vi "mxwScript_API_SetVal_Blob.vi"(7 "itemSelectType":T1, 8 "error in (no error)":errorcluster, 9 "blob":variant, 10 "label":string, 11 "index":i32) -> (0 "error out":errorcluster, 3 "parameter":T2)   [LabVIEW 2017]
uses:
  codeGenAPISupport.llb/cgAPI_mxwScript_Parameter.ctl
  codeGenAPISupport.llb/cgAPI_mxwScript_SetParm_ItemSelectType.ctl
  codeGenAPISupport.llb/cgAPI_mxwScript_SetParm_BlobN.ctl
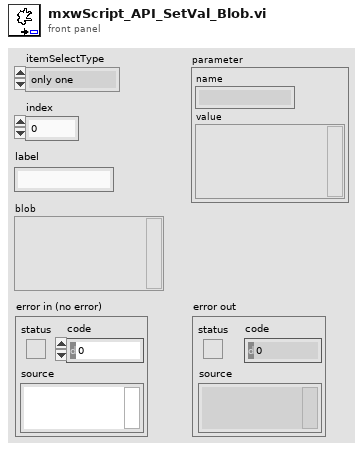
[diagram p1: front panel]
types:
  T1 = typedef "cgAPI_mxwScript_SetParm_ItemSelectType.ctl" = enum16{"only one", "index", "label", "VI name", "legacy"}
  T2 = typedef "cgAPI_mxwScript_Parameter.ctl" = cluster{"name":string, "value":variant}
  T3 = typedef "cgAPI_mxwScript_SetParm_BlobN.ctl" = cluster{"itemSelectType":T1, "index":i32, "label":string, "blob":variant}
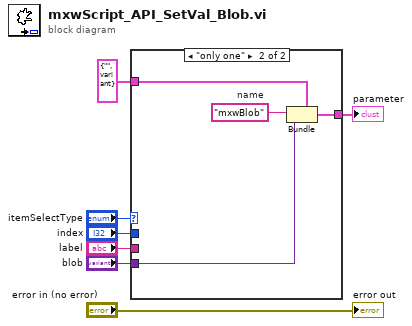
[diagram p0: block diagram]
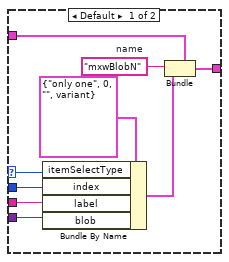
[diagram p2: hidden frame]
diagram:
  n1 = case shown="\"only one\"" "itemSelectType" {
    selector: "itemSelectType" -> [w12 _]
    tunnel: "index" -> [w15 _]
    tunnel: "label" -> [w14 _]
    tunnel: "blob" -> [w13 w17]
    tunnel: T2 {"name"="", "value"=variant} ("parameter") -> [w10 w19]
    tunnel: [w8 w18] -> w1
    frame Default {
      w11 = "mxwBlobN"  # name
      n2 = Bundle By Name(cluster=T3 {"itemSelectType"=enum."only one", "index"=0, "label"="", "blob"=variant} ("codeGenRecipeN"), "itemSelectType"=w12, "index"=w15, "label"=w14, "blob"=w13) -> (w9:T3)
      n3 = Bundle(cluster=w10, "name"=w11, "value"=w9) -> (w8:T2)
    }
    frame "only one" {
      w20 = "mxwBlob"  # name
      n4 = Bundle(cluster=w19, "name"=w20, "value"=w17) -> (w18:T2)
    }
  }
  "parameter" <- w1
  "error out" <- "error in (no error)"
